vi "bats.parser.test.Time.Once.vi"(10 "Expected":T2[](array[typedef])=[{"type"=enum."Time", "side"=0, "orderId "=0, "quantity"=0, "symbol"=0, "price"=0, "executed.qty"=0, "canceled.qty"=0, "remaining.qty"=0, "seconds"=447001, "nanoseconds"=0, "Add"=FALSE, "Edit"=FALSE, "Remove"=FALSE, "seq no"=1, "recv.time"=0, "parse.time"=0}] {"symbol" format="%.0x"; "orderId" format="%.0x"; "side" format="%.0x"}) -> ()   [LabVIEW 2020]
uses:
  Market.Data.Common/fpga/orderbook.command.ctl
  Market.Data.Common/fpga/orderbook.command.type.ctl
  pitch/Time/Time.Parameters.ctl
  Market.Data.Common/fpga/fpganow.common.fpga.lvlib
  pitch/Time/Time.lvclass
panel:
  out "Orderbook.Command[str]":string[](array[string])
  in  "Time.Parameters":T1={"Time"=447001}
  out "Debug":u64[](array[numeric]) format="%.0x"
  out "Passed":bool
  out "OrderBook.Command[]":T2[](array[typedef]) {"symbol" format="%.0x"; "orderId" format="%.0x"; "side" format="%.0x"}
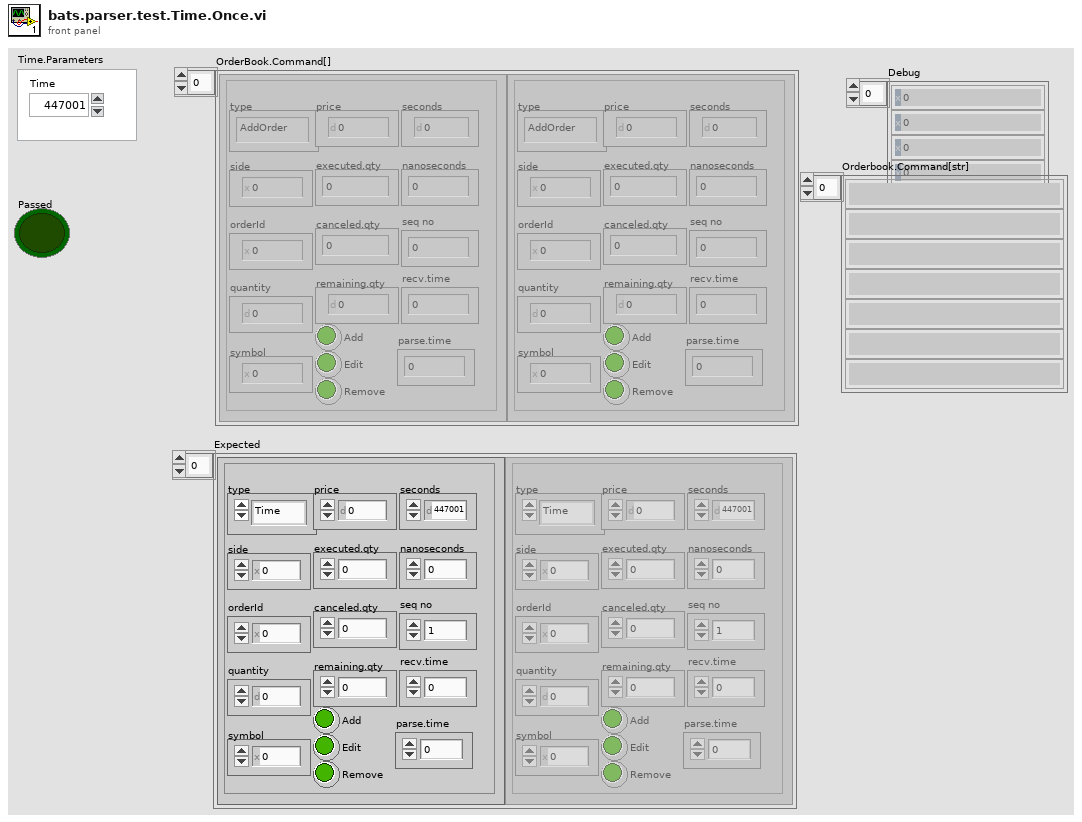
[diagram p1: front panel]
types:
  T1 = typedef "Time.lvclass/Time.Parameters.ctl" = cluster{"Time":u32}
  T2 = typedef "fpganow.common.fpga.lvlib/orderbook.command.ctl" = cluster{"type":T3, "side":u8, "orderId ":u64, "quantity":u32, "symbol":u64, "price":u64, "executed.qty":u32, "canceled.qty":u32, "remaining.qty":u32, "seconds":u64, "nanoseconds":u64, "Add":bool, "Edit":bool, "Remove":bool, "seq no":u32, "recv.time":u64, "parse.time":u64}
  T3 = typedef "fpganow.common.fpga.lvlib/orderbook.command.type.ctl" = enum8{"Time", "AddOrder", "OrderExecuted", "OrderExecutedAtPrice", "ReduceSize", "ModifyOrder", "DeleteOrder", "Get.Everything", "Get.All.Orders", "Get.Top"}
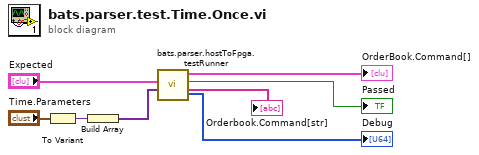
[diagram p0: block diagram]
diagram:
  n1 = To Variant(anything="Time.Parameters") -> (Variant=w3:variant)
  n2 = Build Array(w3) -> (w2:variant[])
  n3 = call "bats.parser.hostToFpga.testRunner.vi"("Test.Messages"=w2, "Expected OrderBook.Command[]"="Expected") -> ("Actual [str]"=→"Orderbook.Command[str]":string[], "Passed"=→"Passed":bool, "OrderBook.Command[]"=→"OrderBook.Command[]":T2[], "Debug"=→"Debug":u64[])  [unwired: 4 in, 2 out]
